vi "displayMessageSender.vi"(8 "error in (no error)":errorcluster, 10 "DatasIN":T1={"PythonSession"=refnum, "Display"=FALSE, "BinThreshold"=0.0, "LIST HOLO BATCH"=[], "Display"=[], "meanHolo"=[], "FEATURES(µm)"=[], "LabelPicture"="", "Status"="", "planeToDisplayFeatures"=enum."XY", "State"=enum."WAIT"}, 11 "QueueMsgIN":refnum<queue>) -> (0 "error out":errorcluster, 2 "DatasOUT":T1={"PythonSession"=refnum, "Display"=FALSE, "BinThreshold"=0.0, "LIST HOLO BATCH"=[], "Display"=[], "meanHolo"=[], "FEATURES(µm)"=[], "LabelPicture"="", "Status"="", "planeToDisplayFeatures"=enum."XY", "State"=enum."WAIT"}, 3 "QueueMsgOut":refnum<queue>)   [LabVIEW 2023]
uses:
  datas.ctl
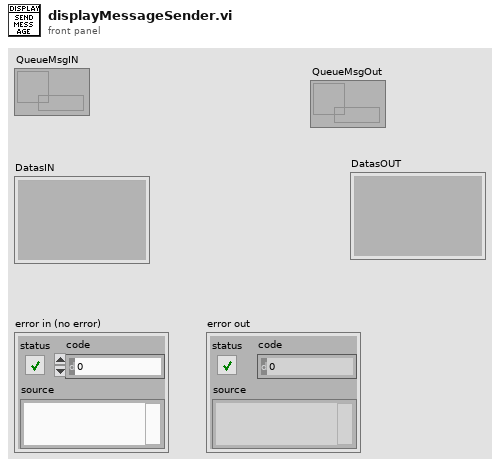
[diagram p1: front panel]
types:
  T1 = typedef "datas.ctl" = cluster{"PythonSession":refnum<k35>, "Display":bool, "BinThreshold":sgl, "LIST HOLO BATCH":path[], "Display":sgl[][], "meanHolo":sgl[][], "FEATURES(µm)":sgl[][], "LabelPicture":string, "Status":string, "planeToDisplayFeatures":enum16{"XY", "XZ", "YZ"}, "State":enum16{"SESSION CLOSED", "WAIT", "TEST WAIT", "TEST IN PROGESS", "BATCH IN PROGRESS"}}
  T2 = enum16{"SESSION CLOSED", "WAIT", "TEST WAIT", "TEST IN PROGESS", "BATCH IN PROGRESS"}
  T3 = cluster{"Holo":sgl[][], "FEATURES(µm)":sgl[][], "planeToDisplayFeatures":enum16{"XY", "XZ", "YZ"}}
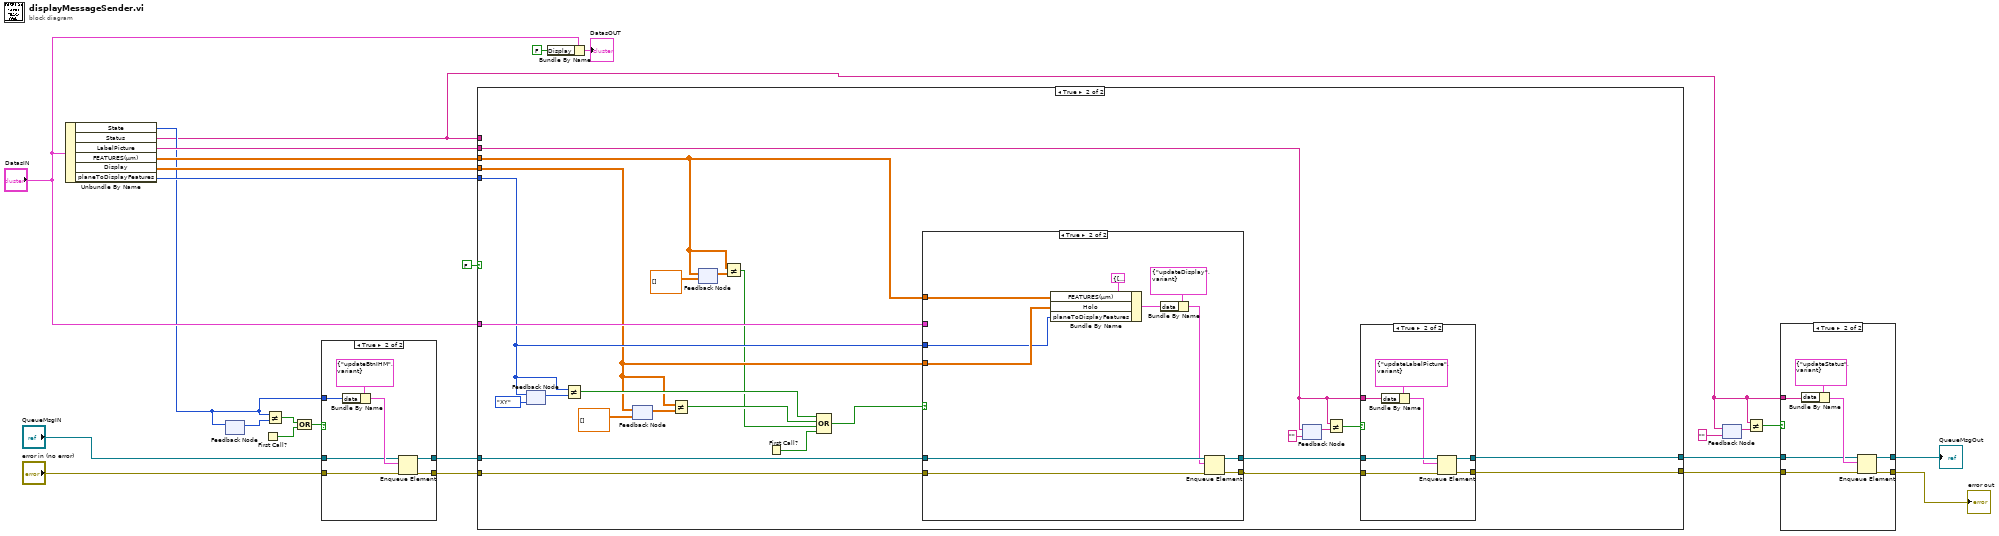
[diagram p0: block diagram]
diagram:
  n1 = Unbundle By Name("DatasIN") -> ("State"=w10:T2, "Status"=w5:string, "LabelPicture"=w25:string, "FEATURES(µm)"=w24:sgl[][], "Display"=w11:sgl[][], "planeToDisplayFeatures"=w12:enum16{"XY", "XZ", "YZ"})
  n2 = feedback #1() -> (w20:T2)  [unwired: 1 in]
  n3 = feedback-in #1(w10) -> ()
  n4 = First Call?() -> (First Call?: T/F=w18:bool)
  n5 = Not Equal?(x=w10, y=w20) -> (x != y?=w19:bool)
  n6 = Compound Arithmetic op=OR(w19, w18) -> (w17:bool)
  n7 = case shown="True" w17 {
    tunnel: w10 -> [_ w32]
    tunnel: "QueueMsgIN" -> [w27 w31]
    tunnel: "error in (no error)" -> [w26 w30]
    tunnel: [w26 w29] -> w14
    tunnel: [w27 w28] -> w13
    frame False {
    }
    frame True {
      n8 = Bundle By Name(cluster=cluster{"command":string, "data":variant} {"command"="updateBtnIHM", "data"=variant} ("element"), "data"=w32) -> (w33:cluster{"command":string, "data":variant})
      n9 = Enqueue Element(queue=w31, element=w33, error in (no error)=w30) -> (queue out=w28:refnum<queue>, error out=w29:errorcluster)  [unwired: 1 in, 1 out]
    }
  }
  n10 = case shown="True" FALSE {
    tunnel: w25 -> [_ w53]
    tunnel: w5 -> [_ _]
    tunnel: [w36 w37] -> w3
    tunnel: [w35 w38] -> w4
    tunnel: w24 -> [_ w47]
    tunnel: "DatasIN" -> [_ w46]
    tunnel: w14 -> [w36 w45]
    tunnel: w13 -> [w35 w44]
    tunnel: w12 -> [_ w43]
    tunnel: w11 -> [_ w42]
    frame False {
    }
    frame True {
      n11 = feedback #2(enum16{"XY", "XZ", "YZ"}."XY" ("planeToDisplayFeatures")) -> (w50:enum16{"XY", "XZ", "YZ"})
      n12 = feedback-in #2(w43) -> ()
      n13 = Not Equal?(x=w43, y=w50) -> (x != y?=w48:bool)
      n14 = feedback #3(sgl[][] [] ("Display")) -> (w60:sgl[][])
      n15 = feedback-in #3(w42) -> ()
      n16 = Not Equal?(x=w42, y=w60) -> (x != y?=w51:bool)
      n17 = feedback #4(sgl[][] [] ("FEATURES")) -> (w59:sgl[][])
      n18 = feedback-in #4(w47) -> ()
      n19 = Not Equal?(x=w47, y=w59) -> (x != y?=w40:bool)
      n20 = First Call?() -> (First Call?: T/F=w41:bool)
      n21 = Compound Arithmetic op=OR(w48, w51, w40, w41) -> (w39:bool)
      n22 = case shown="True" w39 {
        tunnel: w45 -> [w71 w83]
        tunnel: w44 -> [w72 w82]
        tunnel: [w71 w79] -> w54
        tunnel: [w72 w78] -> w55
        tunnel: w42 -> [_ w77]
        tunnel: w47 -> [_ w76]
        tunnel: w46 -> [_ _]
        tunnel: w43 -> [_ w73]
        frame False {
        }
        frame True {
          n23 = Bundle By Name(cluster=T3 {"Holo"=[], "FEATURES(µm)"=[], "planeToDisplayFeatures"=enum."XY"} ("output cluster"), "FEATURES(µm)"=w76, "Holo"=w77, "planeToDisplayFeatures"=w73) -> (w74:T3)
          n24 = Bundle By Name(cluster=cluster{"command":string, "data":variant} {"command"="updateDisplay", "data"=variant} ("element"), "data"=w74) -> (w80:cluster{"command":string, "data":variant})
          n25 = Enqueue Element(queue=w82, element=w80, error in (no error)=w83) -> (queue out=w78:refnum<queue>, error out=w79:errorcluster)  [unwired: 1 in, 1 out]
        }
      }
      n26 = feedback #5("" ("LabelPicture")) -> (w57:string)
      n27 = feedback-in #5(w53) -> ()
      n28 = Not Equal?(x=w53, y=w57) -> (x != y?=w56:bool)
      n29 = case shown="True" w56 {
        tunnel: w54 -> [w62 w70]
        tunnel: w55 -> [w63 w69]
        tunnel: [w62 w66] -> w37
        tunnel: [w63 w65] -> w38
        tunnel: w53 -> [_ w64]
        frame False {
        }
        frame True {
          n30 = Bundle By Name(cluster=cluster{"command":string, "data":variant} {"command"="updateLabelPicture", "data"=variant} ("element"), "data"=w64) -> (w67:cluster{"command":string, "data":variant})
          n31 = Enqueue Element(queue=w69, element=w67, error in (no error)=w70) -> (queue out=w65:refnum<queue>, error out=w66:errorcluster)  [unwired: 1 in, 1 out]
        }
      }
    }
  }
  n32 = Bundle By Name(cluster="DatasIN", "Display"=FALSE) -> (→"DatasOUT":T1)
  n33 = feedback #6("" ("LabelPicture")) -> (w8:string)
  n34 = feedback-in #6(w5) -> ()
  n35 = Not Equal?(x=w5, y=w8) -> (x != y?=w7:bool)
  n36 = case shown="True" w7 {
    tunnel: w5 -> [_ w90]
    tunnel: w4 -> [w85 w89]
    tunnel: w3 -> [w84 w88]
    tunnel: [w84 w87] -> w2
    tunnel: [w85 w86] -> w1
    frame False {
    }
    frame True {
      n37 = Bundle By Name(cluster=cluster{"command":string, "data":variant} {"command"="updateStatus", "data"=variant} ("element"), "data"=w90) -> (w91:cluster{"command":string, "data":variant})
      n38 = Enqueue Element(queue=w89, element=w91, error in (no error)=w88) -> (queue out=w86:refnum<queue>, error out=w87:errorcluster)  [unwired: 1 in, 1 out]
    }
  }
  "error out" <- w2
  "QueueMsgOut" <- w1
